vi "Plotmatrix Format Property.vi"(6 "Update?":bool, 8 "error in (no error)":errorcluster, 9 "Format Property":string[](array[string]), 11 "Single XY Plot In":refnum<vi>) -> (0 "error out":errorcluster, 3 "Single XY Plot Out":refnum<vi>)   [LabVIEW 2017, in "XY Plot Matrix.lvclass"]
uses:
  <vilib>/Math Plots/2D Math Plots/XY Plot Matrix/XY Plot Matrix/XY Plot Matrix.lvclass
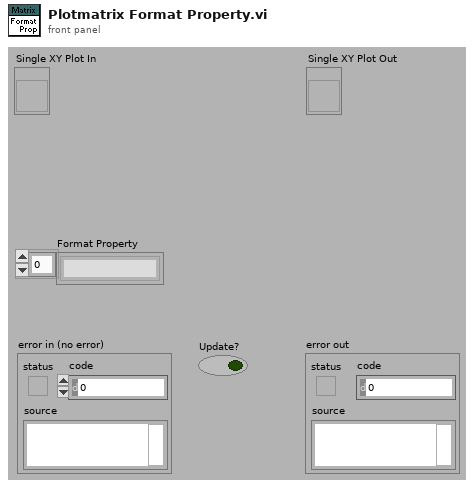
[diagram p1: front panel]
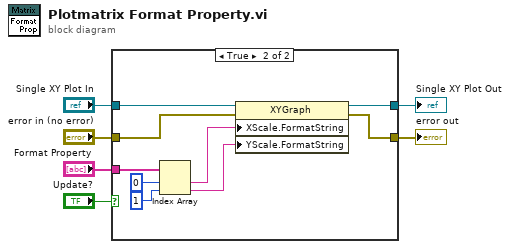
[diagram p0: block diagram]
diagram:
  n1 = case shown="True" "Update?" {
    tunnel: "Format Property" -> [_ w17]
    tunnel: "Single XY Plot In" -> [w8 w14]
    tunnel: [w8 w13] -> w4
    tunnel: "error in (no error)" -> [w7 w12]
    tunnel: [w7 w11] -> w2
    frame False {
    }
    frame True {
      n2 = Index Array(array=w17, index #1=0 ("index"), index #2=1 ("index")) -> (element #1=w16:string, element #2=w15:string)
      n3 = property class="XYGraph"(reference=w14, error in=w12, "XScale.FormatString"=w16, "YScale.FormatString"=w15) -> (reference out=w13:refnum<vi>, error out=w11:errorcluster)
    }
  }
  "Single XY Plot Out" <- w4
  "error out" <- w2
